vi "Task_1.vi"() -> ()   [LabVIEW 2014, in "Diaz_Excercise_3.lvrbt"]
uses:
  Diaz_Excercise_3.lvrbt
  <vilib>/NXT/Dual Mode Library/Display/drawText.vi
panel:
  in  "stop":bool
  out "Distance LED":bool
  out "Wall Proximity":string
  in  "Min Distance":dbl
  in  "Max Distance":dbl
  out "Current Distance":dbl
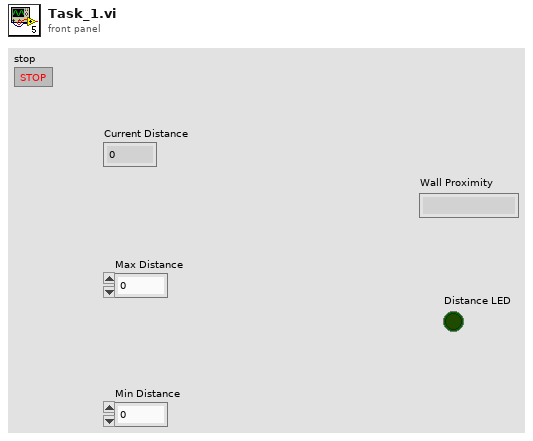
[diagram p1: front panel]
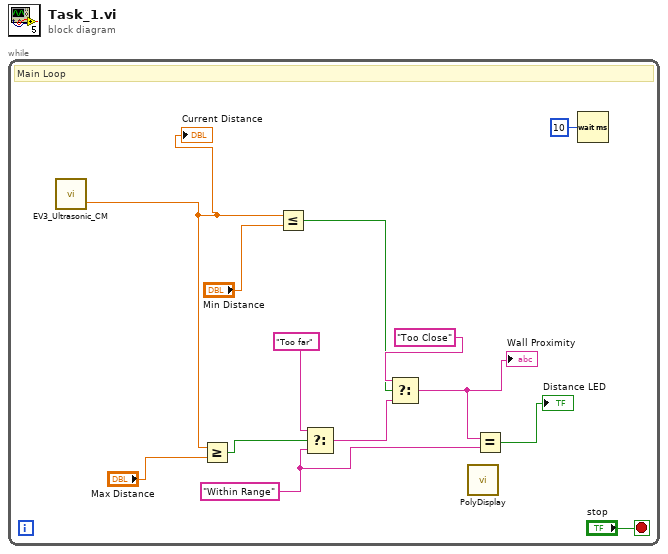
[diagram p0: block diagram]
diagram:
  n1 = while {
    stop <- "stop" stop-if-true
    w8 = "Within Range"
    # "Main Loop"
    n2 = call <vilib>:"EV3_Ultrasonic_CM.vi"() -> ("Centimeters"=w11:sgl)  [unwired: 3 in, 1 out]
    "Current Distance" <- w11
    n3 = Greater Or Equal?(x=w11, y="Max Distance") -> (x >= y?=w10:bool)
    n4 = Less Or Equal?(x=w11, y="Min Distance") -> (x <= y?=w2:bool)
    n5 = Select(t="Too far", s=w10, f=w8) -> (s? t:f=w7:string)
    n6 = Select(t="Too Close", s=w2, f=w7) -> (s? t:f=w3:string)
    "Wall Proximity" <- w3
    n7 = call-poly <vilib>:"PolyDisplay.vi"() -> ()  [unwired: 4 in, 1 out]
    n8 = Equal?(x=w3, y=w8) -> (x = y?=→"Distance LED":bool)
    n9 = Wait (ms)(milliseconds to wait=u32 10) -> ()  [unwired: 1 out]
  }
